vi "SwitchOffAll.vi"(8 "error in (no error)":errorcluster, 11 "LINX Resource":T1) -> (0 "error out":errorcluster, 3 "LINX exit":T1)   [LabVIEW 2018]
uses:
  <vilib>/MakerHub/LINX/Private/Type Defs/LINX Ref.ctl
  <vilib>/MakerHub/LINX/Private/Type Defs/Platform.ctl
  <vilib>/MakerHub/LINX/Private/Type Defs/Interface.ctl
  <vilib>/MakerHub/LINX/Private/Device/Type Defs/LINX Device Config.ctl
  <vilib>/MakerHub/LINX/Private/Device/Type Defs/TCP Config.ctl
  <vilib>/MakerHub/LINX/Private/Device/Type Defs/Channels.ctl
  <vilib>/MakerHub/LINX/LMH-LINX.lvlib
  <vilib>/MakerHub/LINX/Private/Device/Device.lvlib
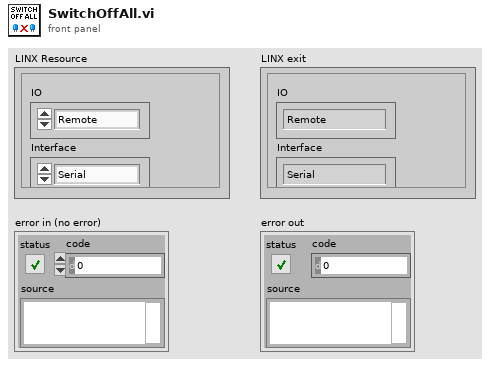
[diagram p1: front panel]
types:
  T1 = typedef "LMH-LINX.lvlib/LINX Ref.ctl" = cluster{"IO":T2, "Interface":T3, "LINX Device Config":T4}
  T2 = typedef "LMH-LINX.lvlib/Platform.ctl" = enum16{"Remote", "Local"}
  T3 = typedef "LMH-LINX.lvlib/Interface.ctl" = enum16{"Serial", "TCP"}
  T4 = typedef "LMH-LINX.lvlib/Device.lvlib/LINX Device Config.ctl" = cluster{"Interface":T3, "COM Port":refnum<visa-resource-name>, "TCP Configuration":T5, "Device Family":u8, "Device ID":u8, "Device Name":string, "TCP Ref":refnum<k5>, "Channels":T6}
  T5 = typedef "LMH-LINX.lvlib/Device.lvlib/TCP Config.ctl" = cluster{"IP Address":string, "Port":u16}
  T6 = typedef "LMH-LINX.lvlib/Channels.ctl" = cluster{"DI":u8[], "DO":u8[], "AI":u8[], "AO":u8[], "PWM":u8[], "QE":u8[], "UART":u8[], "I2C 2":u8[], "SPI":u8[], "CAN":u8[], "Servo":u8[], "AI Ref (V)":dbl, "AI Resolution (Bits)":u8, "AO Ref (V)":dbl, "AO Resolution (Bits)":u8}
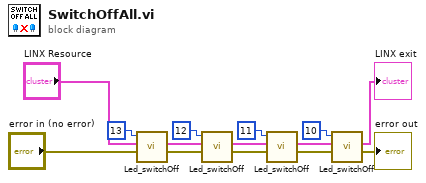
[diagram p0: block diagram]
diagram:
  n1 = call "Led_switchOff.vi"("Error In"="error in (no error)", "LINX Resource"="LINX Resource", "DO Channel"=u8 13) -> ("Error Out"=w2:errorcluster, "LINX exit"=w9:T1)  [unwired: 7 in]
  n2 = call "Led_switchOff.vi"("Error In"=w2, "LINX Resource"=w9, "DO Channel"=u8 12) -> ("Error Out"=w3:errorcluster, "LINX exit"=w10:T1)  [unwired: 7 in]
  n3 = call "Led_switchOff.vi"("Error In"=w3, "LINX Resource"=w10, "DO Channel"=u8 11) -> ("Error Out"=w4:errorcluster, "LINX exit"=w7:T1)  [unwired: 7 in]
  n4 = call "Led_switchOff.vi"("Error In"=w4, "LINX Resource"=w7, "DO Channel"=u8 10) -> ("Error Out"=→"error out":errorcluster, "LINX exit"=→"LINX exit":T1)  [unwired: 7 in]
